vi "PID_Control.vi"(1 "speed(rad/s)":dbl, 2 "kp":dbl, 3 "y":dbl, 4 "r":dbl, 5 "kd":dbl, 6 "ki":dbl) -> (0 "u":dbl)   [LabVIEW 2019]
doc: "Proportional-integral-derivative (PID) controller implemented with the Simulation Module."
uses:
  <vilib>/Simulation/Implementation/Shared/SIMSCR Execution Mode.ctl
  <vilib>/Simulation/Scripting/Companion Diagram/SimConfigNode/SimParams.ctl
  <vilib>/Simulation/Scripting/Companion Diagram/SimConfigNode/_simSolvers.ctl
  <vilib>/Simulation/Param Hierarchy/Typedefs/SIMPH Param Control Actions.ctl
  <vilib>/Simulation/Implementation/Shared/SIM limit type.ctl
  <vilib>/Simulation/Implementation/Shared/NILVSim_ParamChanged.vi
  <vilib>/Simulation/Implementation/Shared/NILVSIM_BeginStep.vi
  <vilib>/Simulation/SignalArithmetic/Implementation/NILVSim Gain.llb/SIM Gain (scalar).vi
  <vilib>/Simulation/ContinuousLinear/Implementation/NILVSim Integrator new.llb/SIM Integrator distributor (scalar).vi
  <vilib>/Simulation/ContinuousLinear/Implementation/NILVSim Integrator new.llb/SIM Integrator collector (scalar).vi
  <vilib>/Simulation/Implementation/Shared/NILVSim_Manager.vi
  <vilib>/Utility/error.llb/Clear Errors.vi
  <vilib>/Simulation/Implementation/Shared/NILVSim_FinalizeModel.vi
  <vilib>/Simulation/Implementation/Shared/SIM Unbundle Sim Info.vi
  <vilib>/Simulation/Implementation/Shared/SIMSH Read Queue.vi
  <vilib>/Simulation/Implementation/Shared/NILVSim_Initialize.vi
  <vilib>/Simulation/Utility/Implementation/NILVSim Get Time and IsAcceptedStep.vi
  <vilib>/Simulation/Implementation/Shared/NILVSim_GetModelError.vi
  <vilib>/Simulation/Implementation/Shared/SIM SimErrorHandler.vi
  <vilib>/Simulation/Implementation/Shared/SIM Bundle Sim Info.vi
  <vilib>/Simulation/Scripting/Companion Diagram/SimConfigNode/SimDog.xnode
  <vilib>/Simulation/Implementation/XNodeFramework/SimXNode/SimX.xnode
  <vilib>/Simulation/ContinuousLinear/Implementation/NILVSim Integrator new.llb/SIM Integrator (scalar).vi
  <vilib>/Simulation/Implementation/Shared/NI_SIM_Implementation.lvlib
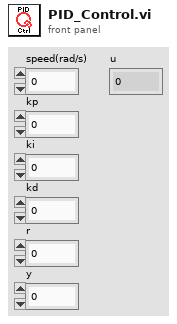
[diagram p1: front panel]
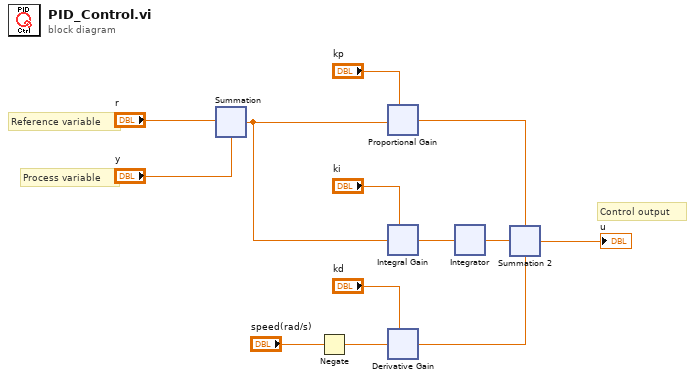
[diagram p0: block diagram]
diagram:
  # "Control output"
  # "Process variable"
  # "Reference variable"
  n1 = xnode ("Summation")("Operand1"="r", "Operand2"="y") -> ("Result"=w3:dbl)
  n2 = Negate(x="speed(rad/s)") -> (-x=w1:dbl)
  n3 = xnode "Proportional Gain"("gain"="kp", "input"=w3) -> ("output"=w10:dbl)  [unwired: 2 in]
  n4 = xnode "Integral Gain"("gain"="ki", "input"=w3) -> ("output"=w8:dbl)  [unwired: 2 in]
  n5 = xnode "Derivative Gain"("gain"="kd", "input"=w1) -> ("output"=w5:dbl)  [unwired: 2 in]
  n6 = xnode ("Integrator")("input"=w8) -> ("output"=w6:dbl)  [unwired: 9 in, 2 out]
  n7 = xnode ("Summation 2")("Operand1"=w10, "Operand2"=w6, "Operand3"=w5) -> ("Result"=→"u":dbl)
